vi "Filepath check and create.vi"(0 "Program Name":string, 1 "Appliance Details":T1, 5 "Wash Temp":string, 7 "Rinse Temp:":string, 9 "LV Program":T3, 11 "Model Family":string, 12 "Model Details Header":string[](array[string])) -> (4 "Model Details Output":string[][](array[string]), 6 "Required Fields":bool, 8 "String":string, 10 "seconds since 1Jan1904":timestamp)   [LabVIEW 2013]
uses:
  Type Definitions/LabView Program.ctl
  Type Definitions/Dishwasher Details.ctl
  <vilib>/Platform/fileVersionInfo.llb/FileVersionInformation.ctl
panel:
  in  "Dishwasher":T4
  in  "Washer":T5
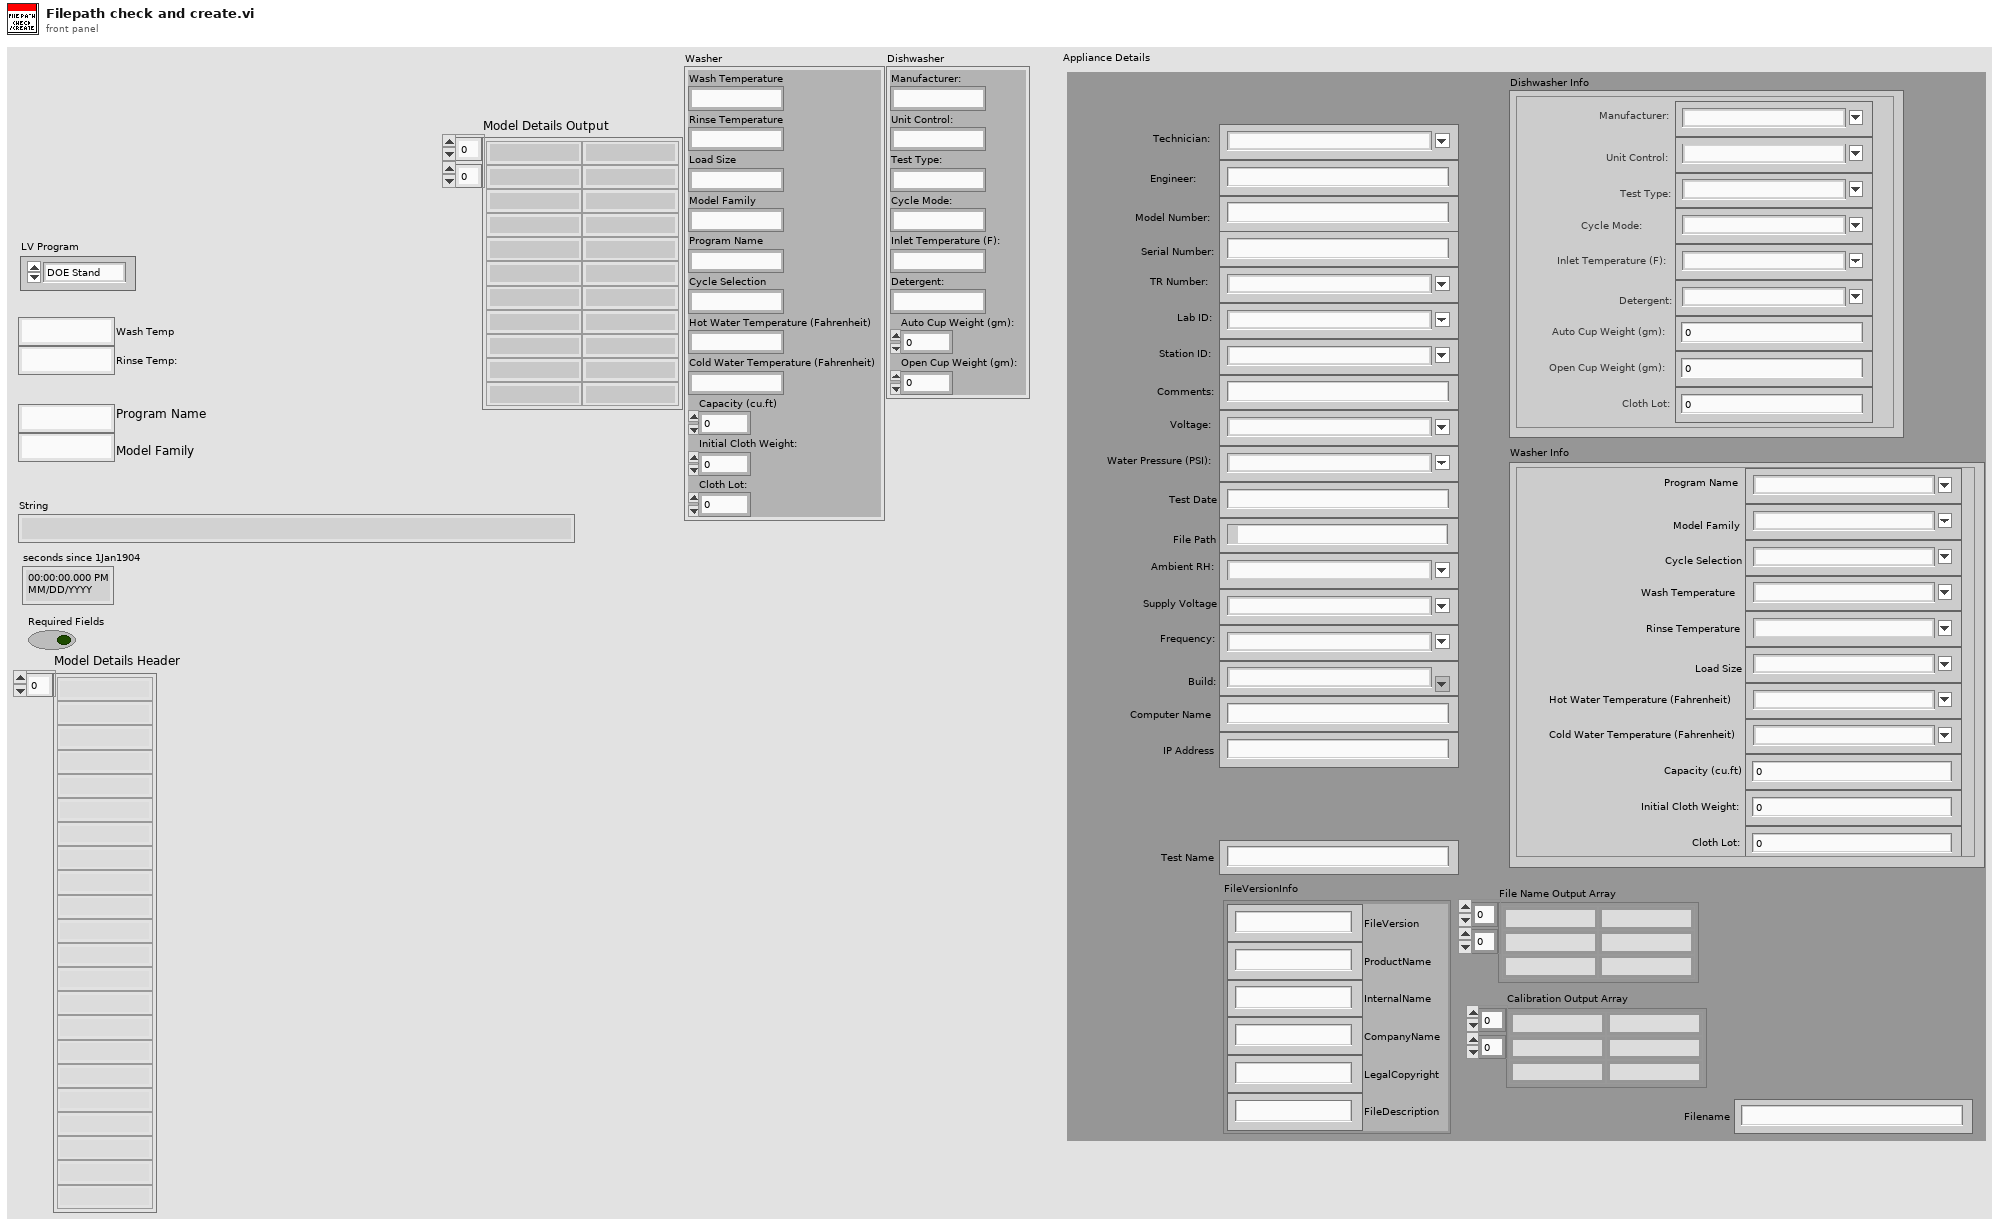
[diagram p1: front panel]
types:
  T1 = typedef "Dishwasher Details.ctl" = cluster{"Engineer:":string, "Model Number:":string, "Serial Number:":string, "Comments:":string, "Station ID:":string, "Technician:":string, "TR Number:":string, "Lab ID:":string, "Voltage:":string, "Water Pressure (PSI):":string, "File Path":path, "FileVersionInfo":T2, "Test Date":string, "Computer Name":string, "IP Address":string, "Test Name":string, "Ambient RH:":string, "Supply Voltage":string, "Frequency:":string, "Build:":string, "Dishwasher Info":cluster{"Cloth Lot:":i32, "Open Cup Weight (gm):":dbl, "Auto Cup Weight (gm):":dbl, "Detergent:":string, "Inlet Temperature (F):":string, "Cycle Mode:":string, "Test Type:":string, "Unit Control:":string, "Manufacturer:":string}, "Washer Info":cluster{"Hot Water Temperature (Fahrenheit)":string, "Cold Water Temperature (Fahrenheit)":string, "Capacity (cu.ft)":dbl, "Initial Cloth Weight:":dbl, "Cloth Lot:":i32, "Model Family":string, "Program Name":string, "Cycle Selection":string, "Wash Temperature":string, "Rinse Temperature":string, "Load Size":string}, "File Name Output Array":string[][], "Calibration Output Array":string[][], "Filename":string}
  T2 = typedef "FileVersionInformation.ctl" = cluster{"FileVersion":string, "ProductName":string, "InternalName":string, "CompanyName":string, "LegalCopyright":string, "FileDescription":string}
  T3 = typedef "LabView Program.ctl" = enum16{"DOE Stand", "Dishwasher Kitchen", "Portable Stand"}
  T4 = cluster{"Manufacturer:":string, "Unit Control:":string, "Test Type:":string, "Cycle Mode:":string, "Inlet Temperature (F):":string, "Detergent:":string, "Auto Cup Weight (gm):":dbl, "Open Cup Weight (gm):":dbl}
  T5 = cluster{"Wash Temperature":string, "Rinse Temperature":string, "Load Size":string, "Model Family":string, "Program Name":string, "Cycle Selection":string, "Hot Water Temperature (Fahrenheit)":string, "Cold Water Temperature (Fahrenheit)":string, "Capacity (cu.ft)":dbl, "Initial Cloth Weight:":dbl, "Cloth Lot:":i32}
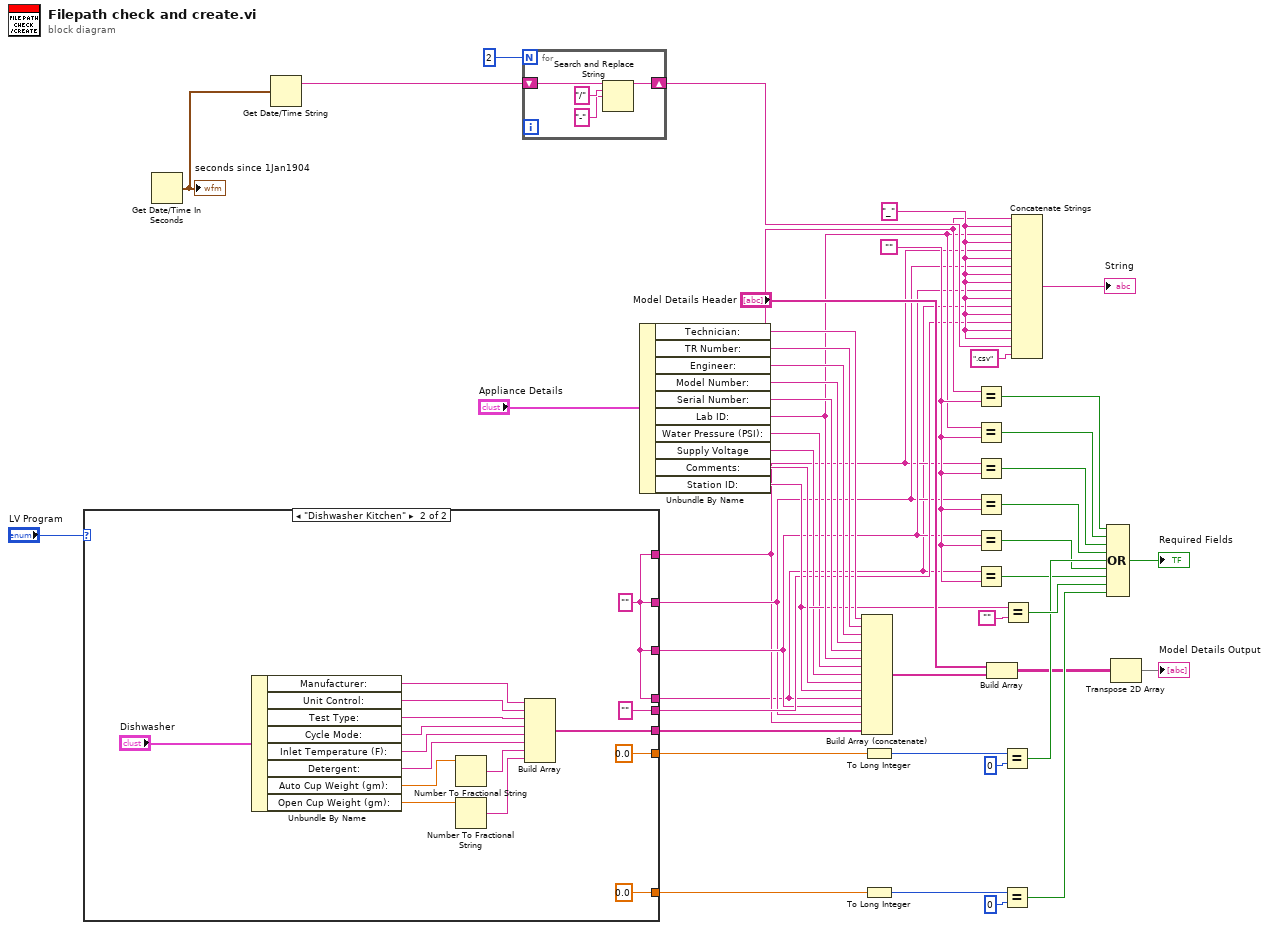
[diagram p0: block diagram]
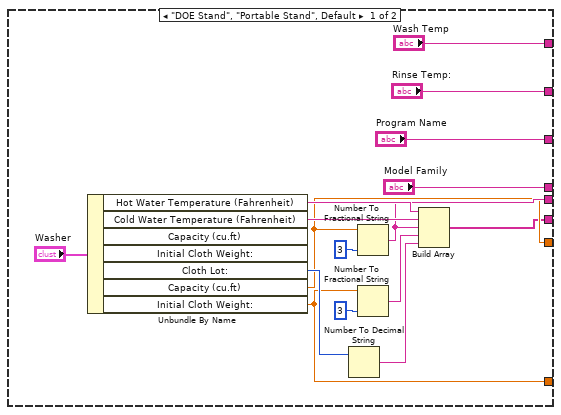
[diagram p2: hidden frame]
diagram:
  w32 = ""
  w46 = "_"
  n1 = case shown="\"Dishwasher Kitchen\"" "LV Program" {
    tunnel: [w57 ""] -> w14
    tunnel: [w55 0.0 ("Initial Cloth Weight:")] -> w12
    tunnel: [w54 0.0 ("Capacity (cu.ft)")] -> w13
    tunnel: [w52 w68] -> w7
    tunnel: ["Program Name" w67] -> w6
    tunnel: ["Rinse Temp:" w67] -> w5
    tunnel: ["Wash Temp" w67] -> w4
    tunnel: ["Model Family" w67] -> w3
    frame "DOE Stand", "Portable Stand", Default {
      n2 = Unbundle By Name("Washer") -> ("Hot Water Temperature (Fahrenheit)"=w59:string, "Cold Water Temperature (Fahrenheit)"=w58:string, "Cloth Lot:"=w60:i32, "Capacity (cu.ft)"=w54:dbl, "Initial Cloth Weight:"=w55:dbl)  [unwired: 2 out]
      n3 = Number To Decimal String(number=w60) -> (decimal integer string=w53:string)  [unwired: 1 in]
      n4 = Number To Fractional String(number=w54, precision (6)=i16 3) -> (F-format string=w57:string)  [unwired: 2 in]
      n5 = Number To Fractional String(number=w55, precision (6)=i16 3) -> (F-format string=w56:string)  [unwired: 2 in]
      n6 = Build Array(w59, w58, w57, w56, w53) -> (w52:string[])
    }
    frame "Dishwasher Kitchen" {
      w67 = "" ("Program Name")
      n7 = Unbundle By Name("Dishwasher") -> ("Manufacturer:"=w78:string, "Unit Control:"=w77:string, "Test Type:"=w76:string, "Cycle Mode:"=w75:string, "Inlet Temperature (F):"=w74:string, "Detergent:"=w73:string, "Auto Cup Weight (gm):"=w72:dbl, "Open Cup Weight (gm):"=w70:dbl)
      n8 = Number To Fractional String(number=w72) -> (F-format string=w71:string)  [unwired: 3 in]
      n9 = Number To Fractional String(number=w70) -> (F-format string=w69:string)  [unwired: 3 in]
      n10 = Build Array(w78, w77, w76, w75, w74, w73, w71, w69) -> (w68:string[])
    }
  }
  n11 = Get Date/Time In Seconds() -> (seconds since 1Jan1904=w33:timestamp)
  "seconds since 1Jan1904" <- w33
  n12 = Get Date/Time String(seconds (now)=w33) -> (date string=w34:string)  [unwired: 2 in, 1 out]
  n13 = for {
    N: 2 -> [_]
    shift-right: [w80] -> w36
    shift-left: w34 -> [w83]
    n14 = Search and Replace String(input string=w83, search string="/", replace string="-" ("replace string (\"\")")) -> (result string=w80:string)  [unwired: 5 in, 3 out]
  }
  n15 = Unbundle By Name("Appliance Details") -> ("Technician:"=w27:string, "TR Number:"=w26:string, "Engineer:"=w25:string, "Model Number:"=w24:string, "Serial Number:"=w23:string, "Lab ID:"=w22:string, "Water Pressure (PSI):"=w16:string, "Supply Voltage"=w15:string, "Comments:"=w21:string, "Station ID:"=w20:string)
  n16 = Build Array (concatenate)(w27, w26, w25, w24, w23, w22, w16, w15, w21, w20, w3, w6, w5, w4, w7) -> (w19:string[])
  n17 = To Long Integer(number=w13) -> (32bit integer=w11:i32)
  n18 = To Long Integer(number=w12) -> (32bit integer=w9:i32)
  n19 = Equal?(x=w26, y=w32) -> (x = y?=w38:bool)
  n20 = Equal?(x=w22, y=w32) -> (x = y?=w39:bool)
  n21 = Equal?(x=w4, y=w32) -> (x = y?=w40:bool)
  n22 = Equal?(x=w5, y=w32) -> (x = y?=w41:bool)
  n23 = Equal?(x=w6, y=w32) -> (x = y?=w31:bool)
  n24 = Equal?(x=w3, y=w32) -> (x = y?=w30:bool)
  n25 = Build Array("Model Details Header", w19) -> (w18:string[][])
  n26 = Equal?(x=w11, y=0) -> (x = y?=w42:bool)
  n27 = Equal?(x=w9, y=0) -> (x = y?=w47:bool)
  n28 = Equal?(x=w20, y="") -> (x = y?=w43:bool)
  n29 = Concatenate Strings(w26, w46, w22, w46, w4, w46, w5, w46, w46, w6, w46, w3, w46, w14, w46, w46, w36, ".csv" ("string")) -> (→"String":string)
  n30 = Compound Arithmetic op=OR(w38, w39, w40, w41, w42, w31, w30, w43, w47) -> (→"Required Fields":bool)
  n31 = Transpose 2D Array(2D array=w18) -> (transposed array=→"Model Details Output":string[][])
